vi "wait.vi"(10 "error in":errorcluster, 11 "wait(ms)":u32) -> (2 "error out":errorcluster)   [LabVIEW 2019]
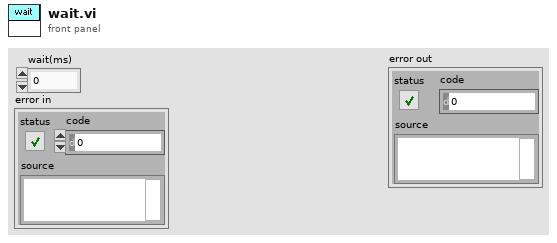
[diagram p1: front panel]
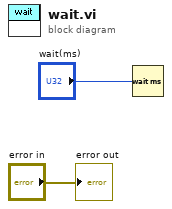
[diagram p0: block diagram]
diagram:
  n1 = Wait (ms)(milliseconds to wait="wait(ms)") -> ()  [unwired: 1 out]
  "error out" <- "error in"
